vi "dfd_Estimate Normalization Order.vi"(8 "error in (no error)":errorcluster, 11 "filter in":T1 {"mSRate_QSettings"."source" items=["Coef a/k"=0, "Coef b/v"=7, "Input"=1, "Output"=2, "Multiplicand"=3, "Product"=4, "Sum"=5, "Delay"=6, "Gain"=8]}) -> (0 "error out":errorcluster, 2 "iteration":i32, 3 "filter out":T1 {"mSRate_QSettings"."source" items=["Coef a/k"=0, "Coef b/v"=7, "Input"=1, "Output"=2, "Multiplicand"=3, "Product"=4, "Sum"=5, "Delay"=6, "Gain"=8]})   [LabVIEW 2017, in "NI_DigFilter_FXP.lvlib"]
uses:
  <vilib>/addons/Digital Filter Design/NI_DigFilter_FXP.lvlib
  <vilib>/addons/Digital Filter Design/_Objects.llb/DFD Filter Obj.ctl
  <vilib>/addons/Digital Filter Design/_Objects.llb/DFD Filter Coef.ctl
  <vilib>/addons/Digital Filter Design/_Objects.llb/DFD Filter Structure Type Selector.ctl
  <vilib>/addons/Digital Filter Design/_Objects.llb/dfd_Internal Quantization Settings.ctl
  <vilib>/addons/Digital Filter Design/_Objects.llb/dfd_Internal Quantization Srcs.ctl
  <vilib>/addons/Digital Filter Design/_Objects.llb/DFD Coef Norm Type.ctl
  <vilib>/Analysis/baseanly.llb/Mean (DBL).vi
  <vilib>/addons/Digital Filter Design/Process.llb/DFD Filtering with State (Array).vi
  <vilib>/addons/Digital Filter Design/NI_DigFilterLicensed.lvlib
  <vilib>/Analysis/NI_AALBase.lvlib
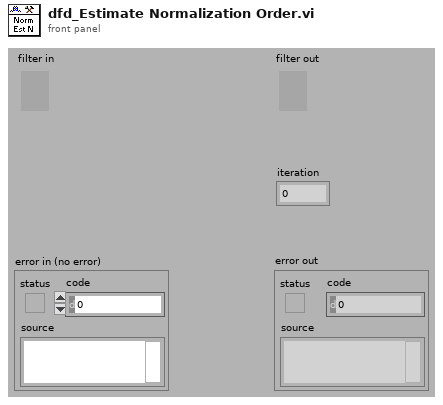
[diagram p1: front panel]
types:
  T1 = typedef "NI_DigFilterLicensed.lvlib/DFD Filter Obj.ctl" = cluster{"mSRate_Fs":dbl, "mSRate_Version":string, "mSRate_Comments":string, "mSRate_OrgCoef":T2, "mSRate_CurCoef":T2, "mSRate_Quantized?":bool, "mSRate_QCoef":T2, "mSRate_QSettings":T4[], "mSRate_Order":i32, "mSRate_Scaling":cluster{"mSRate_ScaleByPowerOf2?":bool, "mSRate_ScaleType":T6}}
  T2 = typedef "NI_DigFilterLicensed.lvlib/DFD Filter Coef.ctl" = cluster{"type":T3, "gain":dbl, "coef a (k)":dbl[], "coef b (v)":dbl[]}
  T3 = typedef "NI_DigFilterLicensed.lvlib/DFD Filter Structure Type Selector.ctl" = enum16{"Undefined", "FIR Direct Form", "FIR Direct Form Transposed", "FIR Symmetric", "FIR Antisymmetric", "IIR Direct Form I", "IIR Direct Form I Transposed", "IIR Direct Form II", "IIR Direct Form II Transposed", "IIR Cascaded Second Order Sections Form I", "IIR Cascaded Second Order Sections Form I Transposed", "IIR Cascaded Second Order Sections Form II", "IIR Cascaded Second Order Sections Form II Transposed", "Lattice Allpass (basic sections)", "Lattice Allpass (one multiplier sections)", "Lattice Allpass (normalized sections)", "Lattice AR (basic sections)", "Lattice AR (one multiplier sections)", "Lattice AR (normalized sections)", "Lattice MA (minimum phase)", "Lattice MA (maximum phase)", "Lattice ARMA (basic sections)", "Lattice ARMA (one multiplier sections)", "Lattice ARMA (normalized sections)"}
  T4 = typedef "NI_DigFilterLicensed.lvlib/dfd_Internal Quantization Settings.ctl" = cluster{"source":T5, "wl":i16, "iwl":i16, "overflow mode":enum16{"Saturation", "Wrap"}, "rounding mode":enum16{"Nearest", "Truncation"}, "signed?":bool}
  T5 = typedef "NI_DigFilterLicensed.lvlib/dfd_Internal Quantization Srcs.ctl" = u16
  T6 = typedef "NI_DigFilterLicensed.lvlib/DFD Coef Norm Type.ctl" = enum16{"No Norm", "Time Domain 1-Norm", "Time Domain 2-Norm", "Time Domain Inf-Norm"}
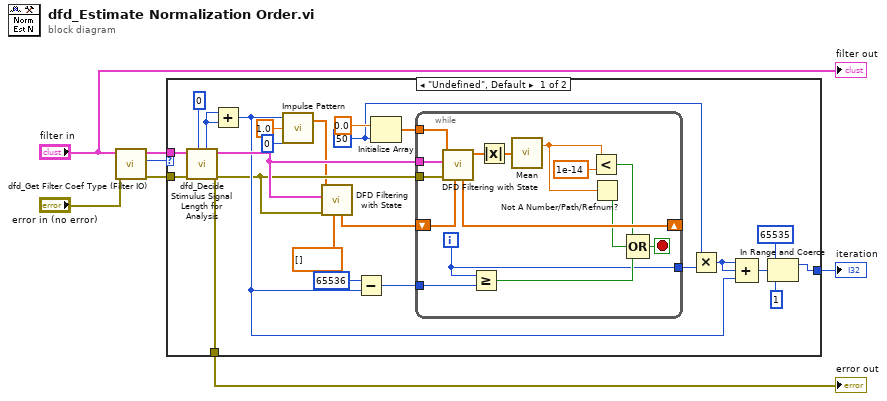
[diagram p0: block diagram]
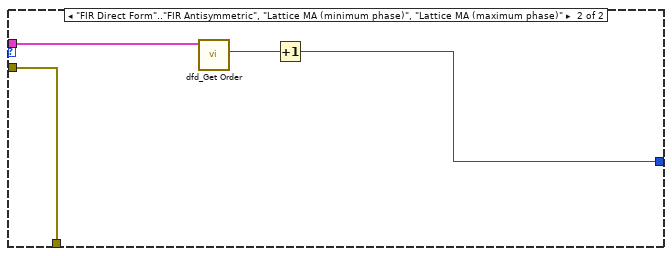
[diagram p2: hidden frame]
diagram:
  n1 = call <vilib>:"dfd_Get Filter Coef Type (Filter IO).vi"("error in (no error)"="error in (no error)", "filter in"="filter in") -> ("error out"=w5:errorcluster, "type"=w4:T3, "filter out"=w3:T1)  [unwired: 1 in, 6 out]
  n2 = case shown="\"Undefined\", Default" w4 {
    tunnel: [w10 w46] -> w2
    tunnel: [w18 w49] -> w7
    tunnel: w3 -> [w29 w48]
    tunnel: w5 -> [w28 w49]
    frame "Undefined", Default {
      w12 = 50 ("dimension size")
      n3 = call <vilib>:"dfd_Decide Stimulus Signal Length for Analysis.vi"("#points in"=0, "error in (no error)"=w28, "filter in"=w29) -> ("error out"=w18:errorcluster, "filter out"=w23:T1, "#points out"=w27:i32)  [unwired: 6 out]
      n4 = Add(x=w27, y=w27) -> (x+y=w19:i32)
      n5 = call <vilib>:"Impulse Pattern.vi"("delay"=0, "amplitude"=1.0, "samples"=w19) -> ("Impulse Pattern"=w17:dbl[])  [unwired: 1 out]
      n6 = call-poly <vilib>:"DFD Filtering with State.vi"("state in"=dbl[] [], "error in (no error)"=w18, "filter"=w23, "signal in"=w17) -> ("state out"=w24:dbl[])  [unwired: 7 out]
      n7 = Subtract(x=65536 ("y"), y=w19) -> (x-y=w25:i32)
      n8 = Initialize Array(0.0 ("element"), w12) -> (w15:dbl[])
      n9 = while {
        tunnel: w23 -> [w36]
        tunnel: w18 -> [w45]
        tunnel: [w38] -> w14
        tunnel: w25 -> [w43]
        shift-right: [w40] -> _
        shift-left: w24 -> [w39]
        tunnel: w15 -> [w37]
        i -> [w38]
        stop <- w42 stop-if-true
        n10 = call-poly <vilib>:"DFD Filtering with State.vi"("state in"=w39, "error in (no error)"=w45, "filter"=w36, "signal in"=w37) -> ("signal out"=w35:dbl[], "state out"=w40:dbl[])  [unwired: 6 out]
        n11 = Greater Or Equal?(x=w38, y=w43) -> (x >= y?=w41:bool)
        n12 = Absolute Value(x=w35) -> (abs(x)=w34:dbl[])
        n13 = call-poly <vilib>:"Mean.vi"("X"=w34) -> ("mean"=w33:dbl)  [unwired: 1 out]
        n14 = Less?(x=w33, y=1e-14) -> (x < y?=w32:bool)
        n15 = Not A Number/Path/Refnum?(number/path/refnum=w33) -> (NaN/Path/Refnum?=w31:bool)
        n16 = Compound Arithmetic op=OR(w32, w31, w41) -> (w42:bool)
      }
      n17 = Multiply(x=w12, y=w14) -> (x*y=w13:i32)
      n18 = Compound Arithmetic op=ADD(w13, w13, w19) -> (w11:i32)
      n19 = In Range and Coerce(upper limit=65535, x=w11, lower limit=1) -> (coerced(x)=w10:i32)  [unwired: 1 out]
    }
    frame "FIR Direct Form".."FIR Antisymmetric", "Lattice MA (minimum phase)", "Lattice MA (maximum phase)" {
      n20 = call <vilib>:"dfd_Get Order.vi"("filter in"=w48) -> ("order"=w47:i32)  [unwired: 1 in, 9 out]
      n21 = Increment(x=w47) -> (x+1=w46:i32)
    }
  }
  "iteration" <- w2
  "error out" <- w7
  "filter out" <- "filter in"
